vi "Get Inside Structure Wires declarations.vi"(11 "GObject in":refnum<vi>) -> (3 "structure inside wires C declarations":string)   [LabVIEW 2014]
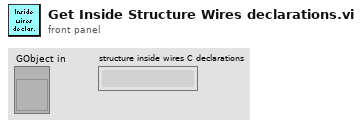
[diagram p1: front panel]
types:
  T1 = cluster{"wire labels":string[], "wire terminals datatypes":string[][]}
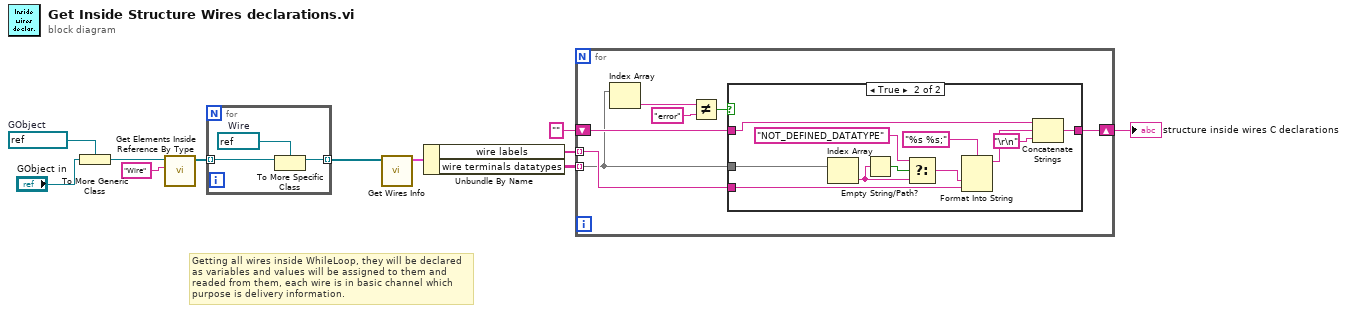
[diagram p0: block diagram]
diagram:
  w2 = refnum<vi> refnum  # GObject
  # "Getting all wires inside WhileLoop, they will be declared as variables and values will be assigned to them and readed from them, each wire is in basic channel which purpose is delivery information."
  n1 = To More Generic Class(target class=w2, reference="GObject in") -> (generic class reference=w3:refnum<vi>)
  n2 = call "Get Elements Inside Reference By Type.vi"("filter element class name"="Wire", "element ref."=w3) -> ("elements ref."=w4:refnum<vi>[])  [unwired: 7 in, 2 out]
  n3 = for {
    tunnel: w4 -> [w13] mode=indexing
    tunnel: [w12] -> w5 mode=indexing
    w14 = refnum<vi> refnum  # Wire
    n4 = To More Specific Class(target class=w14, reference=w13) -> (specific class reference=w12:refnum<vi>)  [unwired: 1 in, 1 out]
  }
  n5 = call "Get Wires Info.vi"("connected\nwires refs."=w5) -> ("output cluster 2"=w8:T1)  [unwired: 10 in]
  n6 = Unbundle By Name(w8) -> ("wire labels"=w6:string[], "wire terminals datatypes"=w7:string[][])
  n7 = for {
    tunnel: w6 -> [w19] mode=indexing
    tunnel: w7 -> [w17] mode=indexing
    shift-right: [w21] -> w10
    shift-left: "" -> [w20]
    n8 = Index Array(array=w17) -> (element=w16:string)  [unwired: 1 in]
    n9 = Not Equal?(x=w16, y="error") -> (x != y?=w15:bool)
    n10 = case shown="True" w15 {
      tunnel: w19 -> [_ w28]
      tunnel: w17 -> [_ w27]
      tunnel: [w22 w25] -> w21
      tunnel: w20 -> [w22 w24]
      frame False {
      }
      frame True {
        n11 = Index Array(array=w27) -> (element=w31:string)  [unwired: 1 in]
        n12 = Empty String/Path?(string/path=w31) -> (empty?=w30:bool)
        n13 = Select(t="NOT_DEFINED_DATATYPE", s=w30, f=w31) -> (s? t:f=w33:string)
        n14 = Format Into String(format string="%s %s;", w33, w28) -> (resulting string=w23:string)  [unwired: 2 in, 1 out]
        n15 = Concatenate Strings(w24, w23, "\r\n") -> (w25:string)
      }
    }
  }
  "structure inside wires C declarations" <- w10
